vi "PH_ImageOperator.PC Read Cali Data.vi"(0 "i ref in":refnum<vi>, 5 "error in (no error)":errorcluster) -> (14 "i ref out":refnum<vi>, 19 "error out":errorcluster)   [LabVIEW 2014, in "PH_ImageOperator.lvlib"]
doc: "This VI reads the calibration data file and sets the own attributes."
uses:
  PH_ImageOperator.lvlib
  PH_ImageCalibrator/PH_ImageCalibrator.Calibration Data.ctl
  PH_StatusHandler/PH_StatusHandler.Status.ctl
  PH_Common/PH_Common.lvlib
  PH_ImageCalibrator/PH_ImageCalibrator.lvlib
  PH_StatusHandler/PH_StatusHandler.lvlib
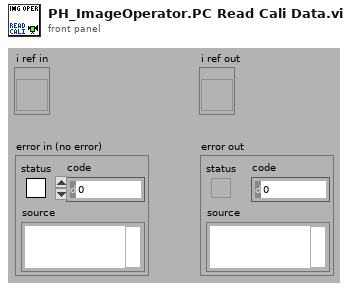
[diagram p1: front panel]
types:
  T1 = typedef "PH_ImageCalibrator.lvlib/PH_ImageCalibrator.Calibration Data.ctl" = cluster{"Date":string, "Time":string, "Cam Settings":cluster{"Cam ID":string, "Gain":dbl, "Brightness":dbl, "Shutter":dbl, "Cam Error":bool, "Mode":i32}, "Background Image":cluster{"Image":dbl[][], "Image Error":bool}, "Linear Calibration":cluster{"Calibration Factor":dbl, "not mm or mrad":bool}, "Energy Calibration":cluster{"Calibration Factor":dbl, "no mJ":bool}}
  T2 = typedef "PH_ImageOperator.lvlib/PH_ImageOperator.i attribute.ctl" = cluster{"GUI Refs":cluster{"Delete":refnum<vi>, "Calibration status":refnum<vi>, "BI subtracted":refnum<vi>, "calc Energy":refnum<vi>, "Energy: expected value":refnum<vi>, "Energy: Tolerance":refnum<vi>, "Energy calculated":refnum<vi>, "Energy":refnum<vi>, "calc Beam Anal":refnum<vi>, "Maj Diam 1/esquare":refnum<vi>, "Min Diam 1/esquare":refnum<vi>, "Azi Angle":refnum<vi>, "Min/Maj Diam esquare":refnum<vi>, "Beam analysed":refnum<vi>, "CoG - x":refnum<vi>, "CoG - y":refnum<vi>, "BA: Method":refnum<vi>, "BA: Steps":refnum<vi>, "BA: Factor":refnum<vi>, "calc Traces":refnum<vi>, "Traces: Fit Gauss":refnum<vi>, "Traces calculated":refnum<vi>, "Maj FWHM":refnum<vi>, "Min FWHM":refnum<vi>, "Major Trace":refnum<vi>, "Minor Trace":refnum<vi>, "Maj Fit Order":refnum<vi>, "Min Fit Order":refnum<vi>, "Position calculated":refnum<vi>, "Position":refnum<vi>, "Type":refnum<vi>, "Center":refnum<vi>, "exp - X":refnum<vi>, "exp - Y":refnum<vi>, "Tolerance":refnum<vi>, "f":refnum<vi>, "M":refnum<vi>, "D":refnum<vi>, "q":refnum<vi>, "Dummy Method":refnum<vi>, "Dummy Type":refnum<vi>, "Global On":refnum<vi>, "Traces: No offset":refnum<vi>, "Maj 99%":refnum<vi>, "Min 99%":refnum<vi>, "GUI FF Image":refnum<vi>, "calc Fill Factor":refnum<vi>, "FF calculated":refnum<vi>, "Fill Factor: Filter?":refnum<vi>, "FF: Damage Threshold":refnum<vi>, "FF: Threshold":refnum<vi>, "FF: max allow. Energy":refnum<vi>, "FF: Fillfactor":refnum<vi>, "Calibration data":refnum<vi>}, "List of GUIs":string[], "Calibration":cluster{"Status":T3, "Calibration data":T1, "Calibration Data File":path}, "Final Image":cluster{"BI Subtraction Failure":bool}, "Energy":cluster{"on":bool, "expected value [mJ]":dbl, "Tolerance [%]":dbl, "State":T3, "Energy [mJ]":dbl, "Unit":string, "calculated @":timestamp}, "Beam Analysis":cluster{"on":bool, "Data":T4, "Method":bool, "Steps":i32, "Factor":i32, "ROI":cluster{"Left":i32, "Top":i32, "Right":i32, "Bottom":i32}, "analysed @":timestamp}, "Trace Analysis":cluster{"on":bool, "Fit on":bool, "Maj FWHM":dbl, "Min FWHM":dbl, "Maj Fit Order":i32, "Min Fit Order":i32, "No Offset":bool, "Maj 99%":dbl, "Min 99%":dbl, "Traces":cluster{"XScaleName":string, "Y Scale Minimum":sgl, "Y Scale Maximum":sgl, "X Scale Minimum":sgl, "X Scale Maximum":sgl, "Traces":cluster{"Index":sgl[], "Trace":dbl[]}[]}[], "analysed @":timestamp}, "Position Analysis":cluster{"on":bool, "exp - X":i32, "exp - Y":i32, "focal length [mm]":dbl, "Magnification":dbl, "Delta":dbl, "Theta":dbl, "Tolerance":dbl, "Type":bool, "analysed @":timestamp}, "Fill Factor":cluster{"on":bool, "Filter on?":bool, "Threshold":dbl, "Damage Threshold [J/cm²]":dbl, "Fillfactor":dbl, "Max. allowed Energy [J]":dbl, "calculated @":timestamp}, "Statistician Service ID":i32, "Images":cluster{"Background":T5, "OP":T5, "GUI":T5, "BA: ROI":T5, "Trace: Turn":T5, "FF: Main":T5, "FF: Help":T5, "PSDB: BG":T5, "PSDB: OP":T5, "PSDB: FF":T5}}
  T3 = typedef "PH_StatusHandler.lvlib/PH_StatusHandler.Status.ctl" = i16
  T4 = typedef "PH_ImageOperator.lvlib/PH_ImageOperator.Beam Analysis Data.ctl" = cluster{"CoG-x":sgl, "CoG-y":sgl, "Maj Dim":dbl, "Min Dim":dbl, "Ellipticity":dbl, "Azimuth Angle [rad]":dbl, "Azi Angle rel to Maj?":bool}
  T5 = typedef "IMAQ Image.ctl" = refnum<image>
  T6 = cluster{"Cam ID":string, "Gain":dbl, "Brightness":dbl, "Shutter":dbl, "Cam Error":bool, "Mode":i32}
  T7 = cluster{"Calibration Factor":dbl, "not mm or mrad":bool}
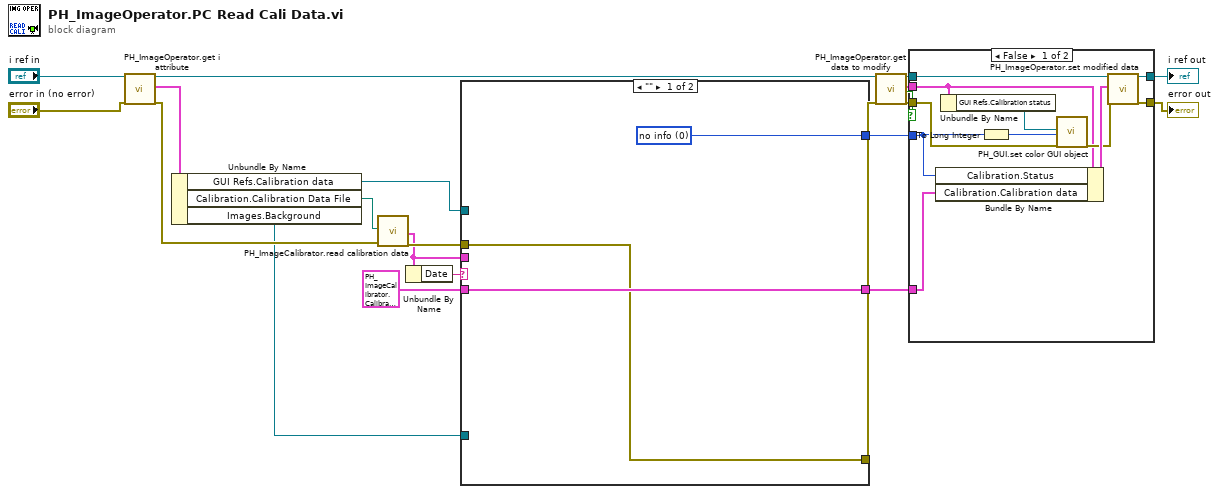
[diagram p0: block diagram]
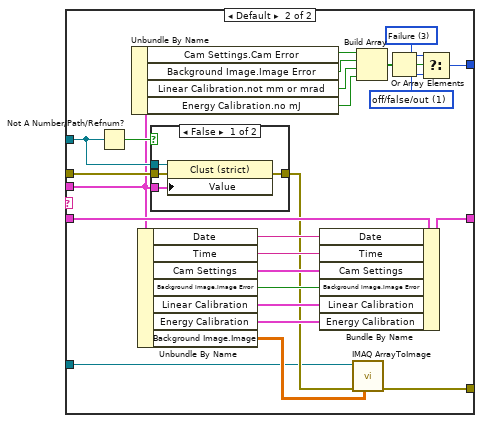
[diagram p3: hidden frame]
diagram:
  n1 = call "PH_ImageOperator.get i attribute.vi"("i ref in"="i ref in", "error in (no error)"="error in (no error)") -> ("i ref out"=w14:refnum<vi>, "i attribute"=w17:T2, "error out"=w18:errorcluster)  [unwired: 15 in]
  n2 = Unbundle By Name(w17) -> ("GUI Refs.Calibration data"=w21:refnum<vi>, "Calibration.Calibration Data File"=w19:path, "Images.Background"=w5:T5)
  n3 = call "PH_ImageCalibrator.read calibration data.vi"("Calibration Data File"=w19, "error in (no error)"=w18) -> ("Calibration data"=w3:T1, "error out"=w20:errorcluster)  [unwired: 16 in]
  n4 = Unbundle By Name(w3) -> ("Date"=w2:string)
  n5 = case shown="\"\"" w2 {
    tunnel: w3 -> [_ w26]
    tunnel: w20 -> [w22 w49]
    tunnel: w21 -> [_ w48]
    tunnel: [w24 w39] -> w7
    tunnel: [w23 w36] -> w6
    tunnel: T1 {"Date"="", "Time"="", "Cam Settings"={"Cam ID"="", "Gain"=0.0, "Brightness"=0.0, "Shutter"=0.0, "Cam Error"=FALSE, "Mode"=0}, "Background Image"={"Image"=[], "Image Error"=FALSE}, "Linear Calibration"={"Calibration Factor"=0.0, "not mm or mrad"=FALSE}, "Energy Calibration"={"Calibration Factor"=0.0, "no mJ"=FALSE}} ("Calibration.Calibration data") -> [w23 w37]
    tunnel: w5 -> [_ w25]
    tunnel: [w22 w28] -> w4
    frame "" {
      w24 = T3 0 items=["no info", "off/false/out", "on/true/in", "Failure", "Alarm", "Status 1", "Status 2", "Status 3"]
    }
    frame Default {
      w38 = T3 3 items=["no info", "off/false/out", "on/true/in", "Failure", "Alarm", "Status 1", "Status 2", "Status 3"] ("t")
      w40 = T3 1 items=["no info", "off/false/out", "on/true/in", "Failure", "Alarm", "Status 1", "Status 2", "Status 3"]
      n6 = Not A Number/Path/Refnum?(number/path/refnum=w48) -> (NaN/Path/Refnum?=w47:bool)
      n7 = Unbundle By Name(w26) -> ("Cam Settings.Cam Error"=w46:bool, "Background Image.Image Error"=w45:bool, "Linear Calibration.not mm or mrad"=w44:bool, "Energy Calibration.no mJ"=w43:bool)
      n8 = Unbundle By Name(w26) -> ("Date"=w35:string, "Time"=w34:string, "Cam Settings"=w33:T6, "Background Image.Image Error"=w32:bool, "Linear Calibration"=w31:T7, "Energy Calibration"=w30:cluster{"Calibration Factor":dbl, "no mJ":bool}, "Background Image.Image"=w27:dbl[][])
      n9 = case shown="False" w47 {
        tunnel: w49 -> [w53 w54]
        tunnel: [w52 w54] -> w29
        tunnel: w48 -> [w51 _]
        tunnel: w26 -> [w50 _]
        frame False {
          n10 = property class="Clust (strict)"(reference=w51, error in=w53, "Value"=w50) -> (error out=w52:errorcluster)  [unwired: 1 out]
        }
        frame True {
        }
      }
      n11 = Bundle By Name(cluster=w37, "Date"=w35, "Time"=w34, "Cam Settings"=w33, "Background Image.Image Error"=w32, "Linear Calibration"=w31, "Energy Calibration"=w30) -> (w36:T1)
      n12 = call "IMAQ ArrayToImage"("Image Pixels (Float)"=w27, "error in (no error)"=w29, "Image"=w25) -> ("error out"=w28:errorcluster)  [unwired: 7 in, 1 out]
      n13 = Build Array(w46, w45, w44, w43) -> (w42:bool[])
      n14 = Or Array Elements(Boolean array=w42) -> (logical OR=w41:bool)
      n15 = Select(t=w38, s=w41, f=w40) -> (s? t:f=w39:T3)
    }
  }
  n16 = call "PH_ImageOperator.get data to modify.vi"("i ref in"=w14, "error in (no error)"=w4) -> ("i ref out"=w12:refnum<vi>, "i attribute"=w8:T2, "timed out"=w10:bool, "error out"=w13:errorcluster)  [unwired: 14 in]
  n17 = case shown="False" w10 {
    tunnel: w13 -> [w61 w66]
    tunnel: w12 -> [w65 w67]
    tunnel: [w64 w67] -> w11
    tunnel: [w63 w66] -> w9
    tunnel: w8 -> [w59 _]
    tunnel: w7 -> [w57 _]
    tunnel: w6 -> [w56 _]
    frame False {
      n18 = Bundle By Name(cluster=w59, "Calibration.Status"=w57, "Calibration.Calibration data"=w56) -> (w62:T2)
      n19 = Unbundle By Name(w59) -> ("GUI Refs.Calibration status"=w58:refnum<vi>)
      n20 = To Long Integer(number=w57) -> (32bit integer=w55:i32)
      n21 = call "PH_GUI.set color GUI object.vi"("GUI object Ref"=w58, "State"=w55, "error in (no error)"=w61) -> ("error out"=w60:errorcluster)  [unwired: 16 in]
      n22 = call "PH_ImageOperator.set modified data.vi"("i ref in"=w65, "i attribute"=w62, "error in (no error)"=w60) -> ("i ref out"=w64:refnum<vi>, "error out"=w63:errorcluster)  [unwired: 15 in]
    }
    frame True {
    }
  }
  "i ref out" <- w11
  "error out" <- w9
